vi "prep.vi"(8 "error in (no error)":errorcluster, 9 "Coordinate System":enum16{"Cartesian", "Cylindrical", "Spherical"}(ring), 10 "Plot processed data In":T1 caption="Data In", 11 "Surface in":refnum<class "Surface.lvclass">) -> (0 "error out":errorcluster, 2 "Plot processed data Out":T1 caption="Data Out", 3 "Surface out":refnum<class "Surface.lvclass">)   [LabVIEW 2020, in "Surface.lvclass"]
uses:
  <vilib>/Native 3D Graph/classes/Surface/Surface.lvclass
  <vilib>/Native 3D Graph/xcontrol/Processed Data.ctl
  <vilib>/Native 3D Graph/typedefs/plot_rep_array.ctl
  <vilib>/Native 3D Graph/typedefs/plot_rep.ctl
  <vilib>/Native 3D Graph/typedefs/range_cluster.ctl
  <vilib>/Native 3D Graph/typedefs/min_max.ctl
  <vilib>/Native 3D Graph/typedefs/plot_rep_mesh_data.ctl
  <vilib>/Native 3D Graph/classes/Surface/Surface.lvclass/Surface.ctl
  <vilib>/Analysis/coordinate.llb/3D Coordinate Conversion (Scalar).vi
  <vilib>/Native 3D Graph/classes/Base Datatype.lvclass
  <vilib>/Native 3D Graph/xcontrol/3DPC_SurfacePlot.xctl
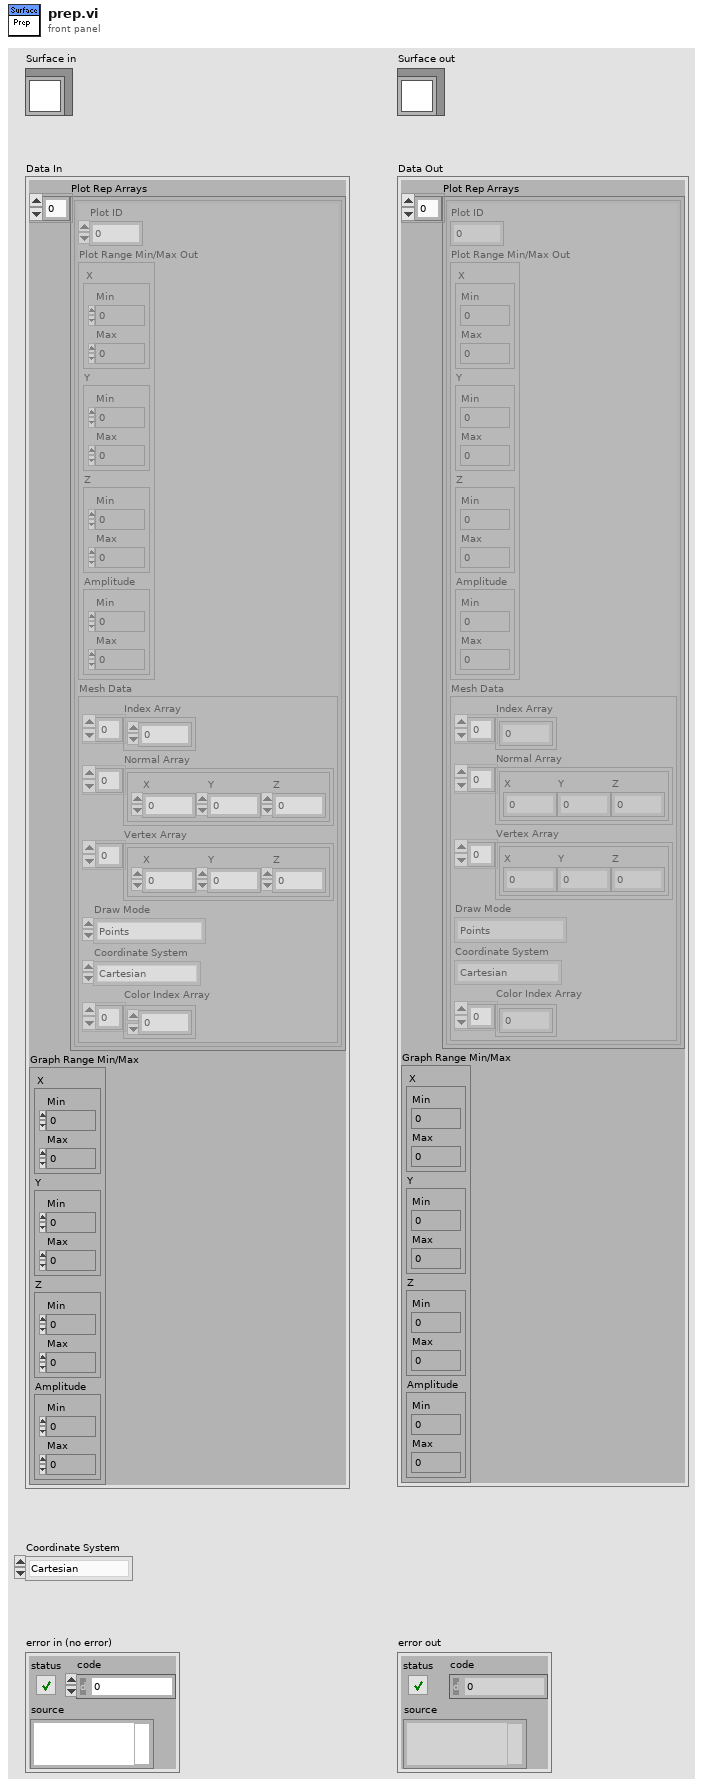
[diagram p1: front panel]
types:
  T1 = typedef "Processed Data.ctl" = cluster{"Plot Rep Arrays":T2, "Graph Range Min/Max":T4}
  T2 = typedef "3DPC_SurfacePlot.xctl/plot_rep_array.ctl" = T3[]
  T3 = typedef "3DPC_SurfacePlot.xctl/plot_rep.ctl" = cluster{"Plot ID":i32, "Plot Range Min/Max Out":T4, "Mesh Data":T6}
  T4 = typedef "3DPC_SurfacePlot.xctl/range_cluster.ctl" = cluster{"X":T5, "Y":T5, "Z":T5, "Amplitude":T5}
  T5 = typedef "3DPC_SurfacePlot.xctl/min_max.ctl" = cluster{"Min":sgl, "Max":sgl}
  T6 = typedef "3DPC_SurfacePlot.xctl/plot_rep_mesh_data.ctl" = cluster{"Index Array":u32[], "Normal Array":cluster{"X":sgl, "Y":sgl, "Z":sgl}[], "Vertex Array":cluster{"X":sgl, "Y":sgl, "Z":sgl}[], "Draw Mode":enum16{"Points", "Lines", "Line Strip", "Line Loop", "Triangles", "Triangle Strip", "Triangle Fan", "Quads", "Quad Strip", "Polygon"}, "Coordinate System":enum16{"Cartesian", "Cylindrical", "Spherical"}, "Color Index Array":i32[]}
  T7 = enum16{"Points", "Lines", "Line Strip", "Line Loop", "Triangles", "Triangle Strip", "Triangle Fan", "Quads", "Quad Strip", "Polygon"}
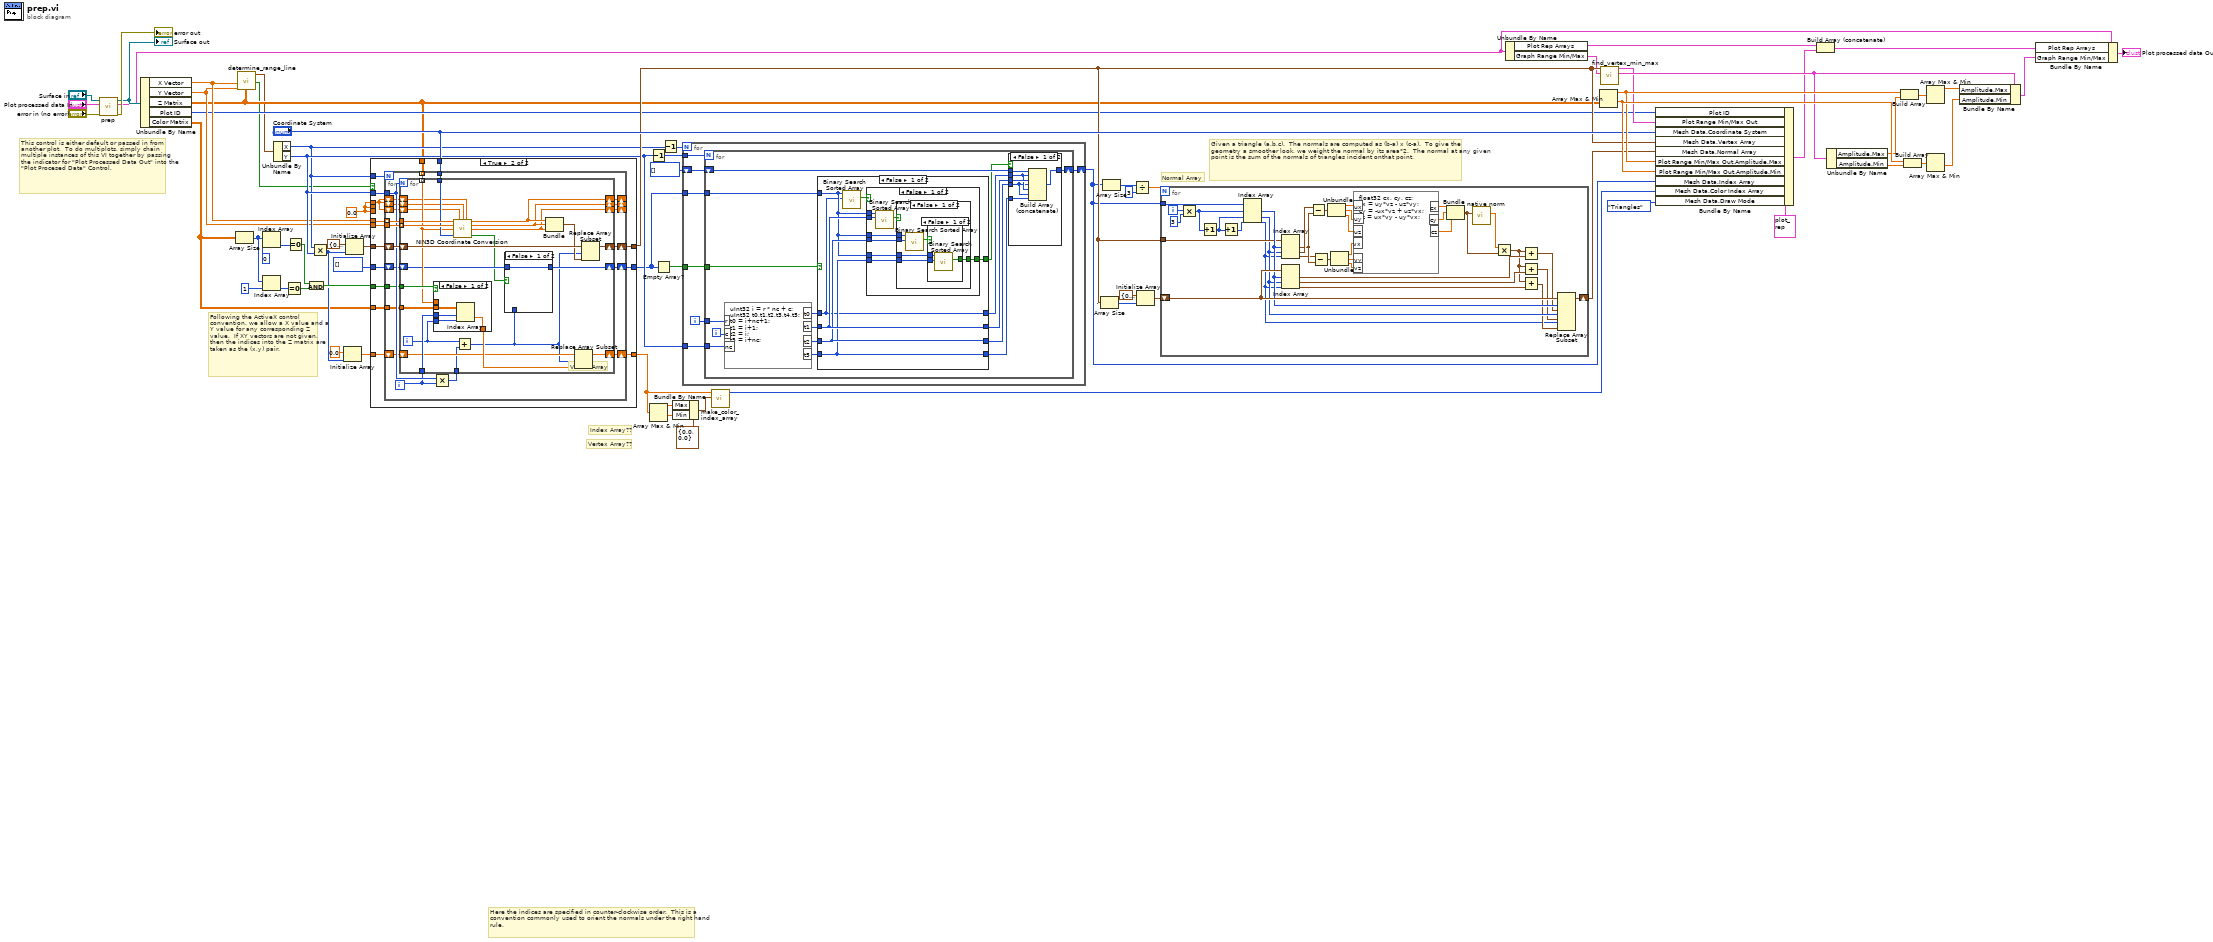
[diagram p0: block diagram]
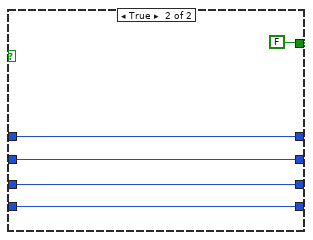
[diagram p5: hidden frame]
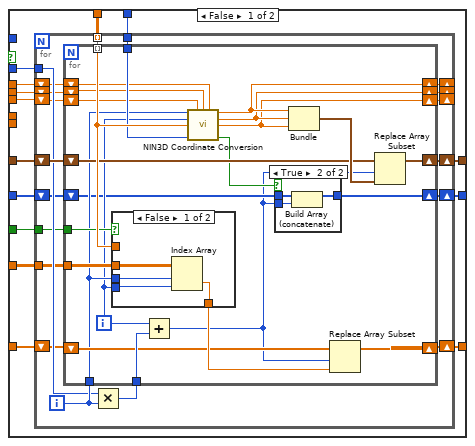
[diagram p7: hidden frame]
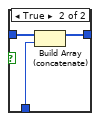
[diagram p10: hidden frame]
diagram:
  w1 = sgl 0.0 ("x")
  # "Following the ActiveX control convention, we allow a X value and a Y value for any corresponding Z value.  If XY vectors are not given, then the indices into the Z matrix are taken as the (x,y) pair."
  # "Given a triangle (a,b,c).  The normals are computed as (b-a) x (c-a).  To give the geometry a smoother look, we weight the normal by its area*2.  The normal at any given point is the sum of the normals of triangles incident onthat point."
  # "Vertex Array??"
  # "Normal Array"
  # "This control is either default or passed in from another plot.  To do multiplots, simply chain multiple instances of this VI together by passing the indicator for \"Plot Processed Data Out\" into the \"Plot Procesed Data\" Control."
  # "Here the indices are specified in counter-clockwise order.  This is a convention commonly used to orient the normals under the right hand rule."
  # "Vertex Array"
  # "Index Array??"
  n1 = call-parent "prep.vi"("error in (no error)"="error in (no error)", "Plot processed data In"="Plot processed data In", "Base Datatype in"="Surface in") -> ("error out"=→"error out":errorcluster, "Plot processed Data Out"=w7:T1, "Base Datatype out"=w66:refnum<class "Surface.lvclass">)  [unwired: 1 in, 5 out]
  "Surface out" <- w66
  n2 = Unbundle By Name(w66) -> ("X Vector"=w11:sgl[], "Y Vector"=w10:sgl[], "Z Matrix"=w4:sgl[][], "Plot ID"=w9:i32, "Color Matrix"=w8:sgl[][])
  n3 = Array Size(array=w8) -> (size(s)=w38:i32[])
  n4 = call <vilib>:"determine_range_line.vi"("Data"=w4, "Y vector"=w10, "X vector"=w11) -> ("Use X/Y vectors?"=w2:bool, "Data Dimension"=w3:cluster{"X":i32, "Y":i32})  [unwired: 2 in, 5 out]
  n5 = Index Array(array=w38, index=0) -> (element=w39:i32)
  n6 = Index Array(array=w38, index=1) -> (element=w40:i32)
  n7 = Unbundle By Name(w3) -> ("X"=w24:i32, "Y"=w50:i32)
  n8 = Equal To 0?(x=w40) -> (x = 0?=w42:bool)
  n9 = Equal To 0?(x=w39) -> (x = 0?=w41:bool)
  n10 = And(x=w41, y=w42) -> (x .and. y?=w43:bool)
  n11 = Multiply(x=w24, y=w50) -> (x*y=w33:i32)
  n12 = Initialize Array(sgl 0.0, w33) -> (w35:sgl[])
  n13 = Initialize Array(cluster{"X":sgl, "Y":sgl, "Z":sgl} {"X"=0.0, "Y"=0.0, "Z"=0.0} ("3D Point"), w33) -> (w25:cluster{"X":sgl, "Y":sgl, "Z":sgl}[])
  n14 = case shown="True" w2 {
    tunnel: w25 -> [w83 w149]
    tunnel: w4 -> [w75 w139]
    tunnel: [w82 w148] -> w56
    tunnel: w24 -> [_ w147]
    tunnel: w50 -> [w81 w146]
    tunnel: w11 -> [_ w145]
    tunnel: w10 -> [_ w144]
    tunnel: "Coordinate System" -> [w77 w143]
    tunnel: w35 -> [w80 w142]
    tunnel: [w79 w138] -> w46
    tunnel: w43 -> [w76 w141]
    tunnel: w8 -> [w78 w140]
    tunnel: u32[] [] -> [w74 w137]
    tunnel: [w73 w136] -> w5
    tunnel: w1 -> [w72 w135]
    tunnel: w1 -> [w71 _]
    tunnel: w1 -> [w70 _]
    frame False {
      n15 = for {
        shift-right: [w101] -> w82
        shift-left: w83 -> [w102]
        tunnel: w75 -> [w100] mode=indexing
        tunnel: w81 -> [w98]
        shift-right: [w95] -> w79
        shift-left: w80 -> [w96]
        tunnel: w78 -> [w94]
        tunnel: w77 -> [w93]
        tunnel: w76 -> [w92]
        shift-right: [w90] -> w73
        shift-left: w74 -> [w91]
        shift-right: [w89] -> _
        shift-left: w72 -> [w86]
        shift-right: [w88] -> _
        shift-left: w71 -> [w85]
        shift-right: [w87] -> _
        shift-left: w70 -> [w84]
        i -> [w99]
        n16 = Multiply(x=w98, y=w99) -> (x*y=w97:i32)
        n17 = for {
          tunnel: w99 -> [w113]
          tunnel: w100 -> [w121] mode=indexing
          shift-right: [w115] -> w101
          shift-left: w102 -> [w120]
          tunnel: w97 -> [w123]
          shift-right: [w116] -> w95
          shift-left: w96 -> [w122]
          tunnel: w94 -> [w119]
          tunnel: w93 -> [w118]
          tunnel: w92 -> [w117]
          shift-right: [w110] -> w90
          shift-left: w91 -> [w111]
          shift-right: [w108] -> w89
          shift-left: w86 -> [w105]
          shift-right: [w107] -> w88
          shift-left: w85 -> [w104]
          shift-right: [w106] -> w87
          shift-left: w84 -> [w103]
          i -> [w112]
          n18 = case shown="False" w117 {
            tunnel: w119 -> [w130 _]
            tunnel: w121 -> [_ w134]
            tunnel: [w133 w134] -> w124
            tunnel: w112 -> [w132 _]
            tunnel: w113 -> [w131 _]
            frame False {
              n19 = Index Array(array=w130, index (row)=w131, index (col)=w132) -> (element=w133:sgl)
            }
            frame True {
            }
          }
          n20 = Add(x=w112, y=w123) -> (x+y=w109:i32)
          n21 = call <vilib>:"NIN3D Coordinate Conversion.vi"("X"=w113, "Z_prev"=w103, "Y_prev"=w104, "X_prev"=w105, "Y"=w112, "Z"=w121, "Coordinate System"=w118) -> ("X out"=w108:sgl, "Y out"=w107:sgl, "Z out"=w106:sgl, "NaN?"=w114:bool)  [unwired: 5 in]
          n22 = case shown="True" w114 {
            tunnel: w111 -> [w126 w129]
            tunnel: [w126 w128] -> w110
            tunnel: w109 -> [_ w127]
            frame False {
            }
            frame True {
              n23 = Build Array (concatenate)(w129, w127) -> (w128:u32[])
            }
          }
          n24 = Bundle("X out"=w108, "Y out"=w107, "Z out"=w106) -> (w125:cluster{"X out":sgl, "Y out":sgl, "Z out":sgl})  [unwired: 1 out]
          n25 = Replace Array Subset(array=w122, new element=w124, index=w109) -> (w116:sgl[])
          n26 = Replace Array Subset(array=w120, new element=w125, index=w109) -> (w115:cluster{"X":sgl, "Y":sgl, "Z":sgl}[])
        }
      }
    }
    frame True {
      n27 = for {
        N: w147 -> [_]
        shift-right: [w169] -> w148
        shift-left: w149 -> [w170]
        tunnel: w139 -> [w168] mode=indexing
        tunnel: w146 -> [w165]
        tunnel: w145 -> [w166] mode=indexing
        tunnel: w144 -> [w167]
        tunnel: w143 -> [w163]
        shift-right: [w161] -> w138
        shift-left: w142 -> [w162]
        tunnel: w141 -> [w160]
        tunnel: w140 -> [w159]
        shift-right: [w156] -> w136
        shift-left: w137 -> [w157]
        shift-right: [w153] -> _
        shift-left: w135 -> [w150]
        shift-right: [w154] -> _
        shift-left: w135 -> [w151]
        shift-right: [w155] -> _
        shift-left: w135 -> [w152]
        i -> [w158]
        n28 = Multiply(x=w165, y=w158) -> (x*y=w164:i32)
        n29 = for {
          N: w165 -> [_]
          tunnel: w168 -> [w188] mode=indexing
          shift-right: [w194] -> w169
          shift-left: w170 -> [w195]
          tunnel: w167 -> [w192] mode=indexing
          tunnel: w166 -> [w193]
          tunnel: w164 -> [w180]
          tunnel: w163 -> [w191]
          shift-right: [w184] -> w161
          shift-left: w162 -> [w185]
          tunnel: w160 -> [w190]
          tunnel: w159 -> [w189]
          tunnel: w158 -> [w187]
          shift-right: [w178] -> w156
          shift-left: w157 -> [w182]
          shift-right: [w174] -> w153
          shift-left: w150 -> [w171]
          shift-right: [w175] -> w154
          shift-left: w151 -> [w172]
          shift-right: [w176] -> w155
          shift-left: w152 -> [w173]
          i -> [w179]
          n30 = case shown="False" w190 {
            tunnel: w189 -> [w203 _]
            tunnel: w188 -> [_ w204]
            tunnel: [w202 w204] -> w186
            tunnel: w179 -> [w201 _]
            tunnel: w187 -> [w200 _]
            frame False {
              n31 = Index Array(array=w203, index (row)=w200, index (col)=w201) -> (element=w202:sgl)
            }
            frame True {
            }
          }
          n32 = call <vilib>:"NIN3D Coordinate Conversion.vi"("X"=w193, "Z_prev"=w171, "Y_prev"=w172, "X_prev"=w173, "Y"=w192, "Z"=w188, "Coordinate System"=w191) -> ("X out"=w176:sgl, "Y out"=w175:sgl, "Z out"=w174:sgl, "NaN?"=w181:bool)  [unwired: 5 in]
          n33 = Add(x=w179, y=w180) -> (x+y=w177:i32)
          n34 = case shown="False" w181 {
            tunnel: w182 -> [w196 w199]
            tunnel: [w196 w198] -> w178
            tunnel: w177 -> [_ w197]
            frame False {
            }
            frame True {
              n35 = Build Array (concatenate)(w199, w197) -> (w198:u32[])
            }
          }
          n36 = Bundle("X out"=w176, "Y out"=w175, "Z out"=w174) -> (w183:cluster{"X out":sgl, "Y out":sgl, "Z out":sgl})  [unwired: 1 out]
          n37 = Replace Array Subset(array=w185, new element=w186, index=w177) -> (w184:sgl[])
          n38 = Replace Array Subset(array=w195, new element=w183, index=w177) -> (w194:cluster{"X":sgl, "Y":sgl, "Z":sgl}[])
        }
      }
    }
  }
  n39 = Decrement(x=w50) -> (x-1=w49:i32)
  n40 = Array Max & Min(array=w46) -> (max value=w52:sgl, min value=w53:sgl)  [unwired: 2 out]
  n41 = Empty Array?(array=w5) -> (empty?=w64:bool)
  n42 = Decrement(x=w24) -> (x-1=w48:i32)
  n43 = Bundle By Name(cluster=T5 {"Min"=0.0, "Max"=0.0} ("Amplitude"), "Max"=w52, "Min"=w53) -> (w45:T5)
  n44 = for {
    N: w48 -> [_]
    shift-right: [w209] -> w54
    shift-left: u32[] [] ("Indices") -> [w211]
    tunnel: w49 -> [w207]
    tunnel: w50 -> [w210]
    tunnel: w5 -> [w206]
    tunnel: w64 -> [w205]
    i -> [w208]
    n45 = for {
      N: w207 -> [_]
      tunnel: w208 -> [w225]
      tunnel: w210 -> [w227]
      shift-right: [w215] -> w209
      shift-left: w211 -> [w226]
      tunnel: w206 -> [w213]
      tunnel: w205 -> [w212]
      i -> [w224]
      n46 = formula code="uInt32 i = r * nc + c; \nuInt32 t0,t1,t2,t3,t4,t5;\nt0 = i+nc+1; \nt1 = i+1; \nt2 = i; \nt5 = i+nc;"("r"=w225, "nc"=w227, "c"=w224) -> ("t0"=w223:u32, "t1"=w221:u32, "t2"=w219:u32, "t5"=w217:u32)
      n47 = case shown="False" w212 {
        tunnel: w213 -> [w231 _]
        tunnel: w223 -> [w229 w259]
        tunnel: [w229 w259] -> w222
        tunnel: w221 -> [w233 w258]
        tunnel: [w233 w258] -> w220
        tunnel: w219 -> [w232 w257]
        tunnel: [w232 w257] -> w218
        tunnel: w217 -> [w230 w256]
        tunnel: [w230 w256] -> w216
        tunnel: [w234 FALSE] -> w214
        frame False {
          n48 = call <vilib>:"Binary Search Sorted Array.vi"("Element"=w229, "Sorted Array"=w231) -> ("Found?"=w228:bool)  [unwired: 9 in]
          n49 = case shown="False" w228 {
            selector: w228 -> [_ w254]
            tunnel: [w241 w254] -> w234
            tunnel: w231 -> [w242 _]
            tunnel: w233 -> [w236 _]
            tunnel: w231 -> [w240 _]
            tunnel: w232 -> [w239 _]
            tunnel: w231 -> [w238 _]
            tunnel: w230 -> [w237 _]
            frame False {
              n50 = call <vilib>:"Binary Search Sorted Array.vi"("Element"=w236, "Sorted Array"=w242) -> ("Found?"=w235:bool)  [unwired: 9 in]
              n51 = case shown="False" w235 {
                selector: w235 -> [_ w253]
                tunnel: [w247 w253] -> w241
                tunnel: w240 -> [w248 _]
                tunnel: w239 -> [w243 _]
                tunnel: w238 -> [w246 _]
                tunnel: w237 -> [w245 _]
                frame False {
                  n52 = call <vilib>:"Binary Search Sorted Array.vi"("Element"=w243, "Sorted Array"=w248) -> ("Found?"=w244:bool)  [unwired: 9 in]
                  n53 = case shown="False" w244 {
                    selector: w244 -> [_ w252]
                    tunnel: [w250 w252] -> w247
                    tunnel: w246 -> [w251 _]
                    tunnel: w245 -> [w249 _]
                    frame False {
                      n54 = call <vilib>:"Binary Search Sorted Array.vi"("Element"=w249, "Sorted Array"=w251) -> ("Found?"=w250:bool)  [unwired: 9 in]
                    }
                    frame True {
                    }
                  }
                }
                frame True {
                }
              }
            }
            frame True {
            }
          }
        }
        frame True {
        }
      }
      n55 = case shown="False" w214 {
        tunnel: w226 -> [w265 w266]
        tunnel: [w264 w266] -> w215
        tunnel: w222 -> [w261 _]
        tunnel: w220 -> [w262 _]
        tunnel: w218 -> [w260 _]
        tunnel: w216 -> [w263 _]
        frame False {
          n56 = Build Array (concatenate)(w265, w261, w262, w260, w261, w260, w263) -> (w264:u32[])
        }
        frame True {
        }
      }
    }
  }
  n57 = call <vilib>:"make_color_index_array.vi"("Amplitude Min/Max"=w45, "Z array"=w46) -> ("Color Index Array"=w55:i32[])  [unwired: 9 out]
  n58 = Array Size(array=w56) -> (size(s)=w12:i32)
  n59 = Array Size(array=w54) -> (size(s)=w16:i32)
  n60 = Divide(x=w16, y=3) -> (x/y=w15:dbl)
  n61 = Initialize Array(cluster{"X":sgl, "Y":sgl, "Z":sgl} {"X"=0.0, "Y"=0.0, "Z"=0.0} ("3D Point"), w12) -> (w13:cluster{"X":sgl, "Y":sgl, "Z":sgl}[])
  n62 = for {
    N: w15 -> [_]
    shift-right: [w294] -> w18
    shift-left: w13 -> [w296]
    tunnel: w54 -> [w299]
    tunnel: w56 -> [w292]
    i -> [w301]
    n63 = Multiply(x=w301, y=3) -> (x*y=w298:i32)
    n64 = Increment(x=w298) -> (x+1=w293:i32)
    n65 = Increment(x=w293) -> (x+1=w297:i32)
    n66 = Index Array(array=w299, index #1=w298, index #2=w293, index #3=w297) -> (element #1=w295:u32, element #2=w291:u32, element #3=w279:u32)
    n67 = Index Array(array=w292, index #1=w295, index #2=w291, index #3=w279) -> (element #1=w289:cluster{"X":sgl, "Y":sgl, "Z":sgl}, element #2=w290:cluster{"X":sgl, "Y":sgl, "Z":sgl}, element #3=w282:cluster{"X":sgl, "Y":sgl, "Z":sgl})
    n68 = Index Array(array=w296, index #1=w295, index #2=w291, index #3=w279) -> (element #1=w288:cluster{"X":sgl, "Y":sgl, "Z":sgl}, element #2=w287:cluster{"X":sgl, "Y":sgl, "Z":sgl}, element #3=w285:cluster{"X":sgl, "Y":sgl, "Z":sgl})
    n69 = Subtract(x=w290, y=w289) -> (x-y=w278:cluster{"X":sgl, "Y":sgl, "Z":sgl})
    n70 = Subtract(x=w282, y=w289) -> (x-y=w274:cluster{"X":sgl, "Y":sgl, "Z":sgl})
    n71 = Unbundle(w278) -> ("X"=w277:sgl, "Y"=w276:sgl, "Z"=w275:sgl)
    n72 = Unbundle(w274) -> ("X"=w273:sgl, "Y"=w272:sgl, "Z"=w271:sgl)
    n73 = formula code="float32 cx, cy, cz;\ncx = uy*vz - uz*vy;\ncy = -ux*vz + uz*vx;\ncz = ux*vy - uy*vx;"("ux"=w277, "uy"=w276, "uz"=w275, "vx"=w273, "vy"=w272, "vz"=w271) -> ("cx"=w270:sgl, "cy"=w269:sgl, "cz"=w268:sgl)
    n74 = Bundle(w270, w269, w268) -> (w267:cluster{sgl, sgl, sgl})  [unwired: 1 in]
    n75 = call <vilib>:"native norm.vi"("Vector"=w267) -> ("Norm"=w280:sgl)  [unwired: 10 in]
    n76 = Multiply(x=w280, y=w267) -> (x*y=w286:cluster{sgl, sgl, sgl})
    n77 = Add(x=w286, y=w288) -> (x+y=w281:cluster{sgl, sgl, sgl})
    n78 = Add(x=w286, y=w287) -> (x+y=w284:cluster{sgl, sgl, sgl})
    n79 = Add(x=w286, y=w285) -> (x+y=w283:cluster{sgl, sgl, sgl})
    n80 = Replace Array Subset(array=w296, new element #1=w281, index #1=w295, new element #2=w284, index #2=w291, new element #3=w283, index #3=w279) -> (w294:cluster{"X":sgl, "Y":sgl, "Z":sgl}[])
  }
  n81 = Unbundle By Name(w7) -> ("Plot Rep Arrays"=w19:T2, "Graph Range Min/Max"=w26:T4)
  n82 = Array Max & Min(array=w4) -> (max value=w60:sgl, min value=w62:sgl)  [unwired: 2 out]
  n83 = call <vilib>:"find_vertex_min_max.vi"("Total Range Min/Max"=w26, "Vertex Array"=w56) -> ("Total Range Out"=w29:T4, "This Range Min/Max Out"=w27:T4)  [unwired: 8 out]
  n84 = Bundle By Name(cluster=T3 {"Plot ID"=0, "Plot Range Min/Max Out"={"X"={"Min"=0.0, "Max"=0.0}, "Y"={"Min"=0.0, "Max"=0.0}, "Z"={"Min"=0.0, "Max"=0.0}, "Amplitude"={"Min"=0.0, "Max"=0.0}}, "Mesh Data"={"Index Array"=[], "Normal Array"=[], "Vertex Array"=[], "Draw Mode"=enum."Points", "Coordinate System"=enum."Cartesian", "Color Index Array"=[]}} ("Plot Representation"), "Plot ID"=w9, "Plot Range Min/Max Out"=w27, "Mesh Data.Coordinate System"="Coordinate System", "Mesh Data.Vertex Array"=w56, "Mesh Data.Normal Array"=w18, "Plot Range Min/Max Out.Amplitude.Max"=w60, "Plot Range Min/Max Out.Amplitude.Min"=w62, "Mesh Data.Index Array"=w54, "Mesh Data.Color Index Array"=w55, "Mesh Data.Draw Mode"=T7."Triangles") -> (w20:T3)
  n85 = Build Array (concatenate)(w19, w20) -> (w21:T2)
  n86 = Unbundle By Name(w29) -> ("Amplitude.Max"=w59:sgl, "Amplitude.Min"=w31:sgl)
  n87 = Build Array(w60, w59) -> (w28:sgl[])
  n88 = Build Array(w62, w31) -> (w32:sgl[])
  n89 = Array Max & Min(array=w28) -> (max value=w61:sgl)  [unwired: 3 out]
  n90 = Array Max & Min(array=w32) -> (min value=w63:sgl)  [unwired: 3 out]
  n91 = Bundle By Name(cluster=w29, "Amplitude.Max"=w61, "Amplitude.Min"=w63) -> (w30:T4)
  n92 = Bundle By Name(cluster=w7, "Plot Rep Arrays"=w21, "Graph Range Min/Max"=w30) -> (→"Plot processed data Out":T1)
